vi "Motion_Move Gantry To Position.vi"(5 "Timeout sec (-1 = No timeout)":i32=-1, 7 "Position Tolerance (0.1in)":dbl=0.1, 8 "error in":errorcluster, 10 "Gantry Move Data":T1={"Gantry Accel/Decel"=5.0, "Gantry Velocity"=5.0, "X-Position"=0.0, "Y-Position"=0.0, "Z-Position"=0.0} {"Z-Position" format="%_7g"; "Y-Position" format="%_7g"; "X-Position" format="%_7g"; "Gantry Velocity" format="%_7g"; "Gantry Accel/Decel" format="%_7g"}, 11 "TCP address:port":string="192.168.0.3:502") -> (0 "error out":errorcluster, 2 "elapsed time":dbl[unit]=nan format="%.1f")   [LabVIEW 2010]
uses:
  Motion_Gantry Position.ctl
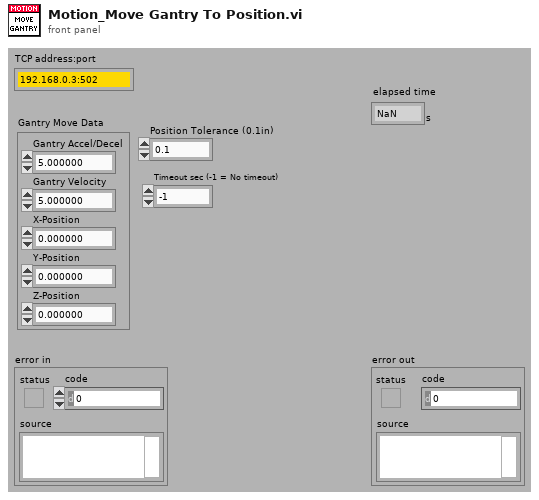
[diagram p1: front panel]
types:
  T1 = typedef "Motion_Gantry Position.ctl" = cluster{"Gantry Accel/Decel":dbl, "Gantry Velocity":dbl, "X-Position":dbl, "Y-Position":dbl, "Z-Position":dbl}
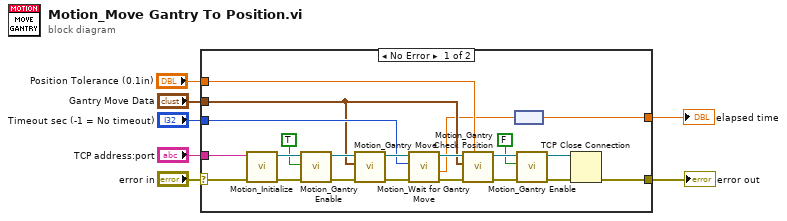
[diagram p0: block diagram]
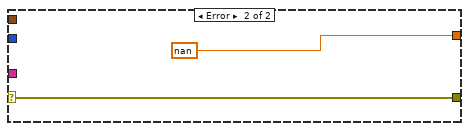
[diagram p2: hidden frame]
diagram:
  n1 = case shown="No Error" "error in" {
    selector: "error in" -> [w27 w31]
    tunnel: [w29 w31] -> w7
    tunnel: "TCP address:port" -> [w28 _]
    tunnel: [w8 dbl[unit] nan ("elapsed time")] -> w4
    tunnel: "Timeout sec (-1 = No timeout)" -> [w16 _]
    tunnel: "Gantry Move Data" -> [w15 _]
    tunnel: "Position Tolerance (0.1in)" -> [w10 _]
    frame No Error {
      n2 = call "Motion_Initialize.vi"("error in (no error)"=w27, "TCP address:port (192.168.0.3:502)"=w28) -> ("error out"=w26:errorcluster, "connection ID"=w25:refnum<k5>)  [unwired: 8 in]
      n3 = call "Motion_Gantry Enable.vi"("error in (no error)"=w26, "Enable? (T)"=TRUE, "TCP Connection Refnum in"=w25) -> ("error out"=w23:errorcluster, "TCP Connection Refnum (dup)"=w24:refnum<k5>)  [unwired: 7 in]
      n4 = call "Motion_Gantry Move.vi"("error in (no error)"=w23, "Gantry Move Data"=w15, "TCP Connection Refnum in"=w24) -> ("error out"=w20:errorcluster, "TCP Connection Refnum (dup)"=w21:refnum<k5>)  [unwired: 7 in]
      n5 = call "Motion_Wait for Gantry Move.vi"("error in (no error)"=w20, "Timeout sec (-1 = No timeout)"=w16, "TCP Connection Refnum in"=w21) -> ("error out"=w18:errorcluster, "Time Elapsed"=w9:dbl, "TCP Connection Refnum (dup)"=w19:refnum<k5>)  [unwired: 5 in, 1 out]
      n6 = call "Motion_Gantry Check Position.vi"("Tolerance (0.1)"=w10, "error in (no error)"=w18, "Gantry Move Data"=w15, "TCP Connection Refnum"=w19) -> ("error out"=w13:errorcluster, "TCP Connection Refnum (dup)"=w17:refnum<k5>)  [unwired: 5 in, 1 out]
      n7 = node(w9) -> (w8:dbl[unit])
      n8 = call "Motion_Gantry Enable.vi"("error in (no error)"=w13, "Enable? (T)"=FALSE, "TCP Connection Refnum in"=w17) -> ("error out"=w11:errorcluster, "TCP Connection Refnum (dup)"=w12:refnum<k5>)  [unwired: 7 in]
      n9 = TCP Close Connection(connection ID=w12, error in (no error)=w11) -> (error out=w29:errorcluster)  [unwired: 1 in, 1 out]
    }
    frame Error {
    }
  }
  "error out" <- w7
  "elapsed time" <- w4
